vi "RampVoltagewithDDSv7.vi"() -> ()   [LabVIEW 2016]
uses:
  <vilib>/DAQmx/write.llb/DAQmx Write (Digital 1D Wfm NChan NSamp).vi
  <vilib>/DAQmx/write.llb/DAQmx Write (Analog 2D DBL NChan NSamp).vi
  <vilib>/DAQmx/create/channels.llb/DAQmx Create Channel (AO-Voltage-Basic).vi
  <vilib>/DAQmx/create/channels.llb/DAQmx Create Channel (DO-Digital Output).vi
  <vilib>/DAQmx/configure/timing.llb/DAQmx Timing (Sample Clock).vi
  <vilib>/DAQmx/configure/trigger.llb/DAQmx Start Trigger (Digital Edge).vi
  <vilib>/DAQmx/miscellaneous.llb/DAQmx Fill In Error Info.vi
  <vilib>/Waveform/DWDTOps.llb/DWDT Boolean Array to Digital.vi
  <vilib>/Waveform/DWDTOps.llb/DWDT Uncompress Digital.vi
  <vilib>/Waveform/DTblOps.llb/DTbl Digital to Analog.vi
  <resource>/objmgr/daqmx.rc
panel:
  in  "Reset Digital Outputs":bool
  in  "DDS Trigger delay (ms)":dbl step=0.01
  in  "DDS Trigger (Port 0 Line 1)":tag="Dev2/port0/line1"
  out "Digital Output":cluster{i32, dbl, dbl[][]}(graph)={0, 1e-05, [[5.0, 5.0, 5.0, 5.0, 5.0, 5.0, 5.0, 5.0, 5.0, 5.0, 5.0, 5.0, 5.0, 5.0, 5.0, 5.0, 5.0, 5.0, 5.0, 5.0, 5.0, 5.0, 5.0, 5.0, 5.0, 5.0, 5.0, 5.0, 5.0, 5.0, 5.0, 5.0, 5.0, 5.0, 5.0, 5.0, 5.0, 5.0, 5.0, 5.0, 5.0, 5.0, 5.0, 5.0, 5.0, 5.0, 5.0, 5.0, 5.0, 5.0, 5.0, 5.0, 5.0, 5.0, 5.0, 5.0, 5.0, 5.0, 5.0, 5.0, 5.0, 5.0, 5.0, 5.0, 5.0, 5.0, 5.0, 5.0, 5.0, 5.0, 5.0, 5.0, 5.0, 5.0, 5.0, 5.0, 5.0, 5.0, 5.0, 5.0, 5.0, 5.0, 5.0, 5.0, 5.0, 5.0, 5.0, 5.0, 5.0, 5.0, 5.0, 5.0, 5.0, 5.0, 5.0, 5.0, 5.0, 5.0, 5.0, 5.0, 0.0, 0.0, 0.0, 0.0, 0.0, 0.0, 0.0, 0.0, 0.0, 0.0, 0.0, 0.0, 0.0, 0.0, 0.0, 0.0, 0.0, 0.0, 0.0, 0.0, 0.0, 0.0, 0.0, 0.0, 0.0, 0.0, 0.0, 0.0, 0.0, 0.0, 0.0, 0.0, 0.0, 0.0, 0.0, 0.0, 0.0, 0.0, 0.0, 0.0, 0.0, 0.0, 0.0, 0.0, 0.0, 0.0, 0.0, 0.0, 0.0, 0.0, 0.0, 0.0, 0.0, 0.0, 0.0, 0.0, 0.0, 0.0, 0.0, 0.0, 0.0, 0.0, 0.0, 0.0, 0.0, 0.0, 0.0, 0.0, 0.0, 0.0, 0.0, 0.0, 0.0, 0.0, 0.0, 0.0, 0.0, 0.0, 0.0, 0.0, 0.0, 0.0, 0.0, 0.0, 0.0, 0.0, 0.0, 0.0, 0.0, 0.0, 0.0, 0.0, 0.0, 0.0, 0.0, 0.0, 0.0, 0.0, 0.0, 0.0, 0.0, 0.0, 0.0, 0.0, 0.0, 0.0, 0.0, 0.0, 0.0, 0.0, 0.0, 0.0, 0.0, 0.0, 0.0, 0.0, 0.0, 0.0, 0.0, 0.0, 0.0, 0.0, 0.0, 0.0, 0.0, 0.0, 0.0, 0.0, 0.0, 0.0, 0.0, 0.0, 0.0, 0.0, 0.0, 0.0, 0.0, 0.0, 0.0, 0.0, 0.0, 0.0, 0.0, 0.0, 0.0, 0.0, 0.0, 0.0, 0.0, 0.0, 0.0, 0.0, 0.0, 0.0, 0.0, 0.0, 0.0, 0.0, 0.0, 0.0, 0.0, 0.0, 0.0, 0.0, 0.0, 0.0, 0.0, 0.0, 0.0, 0.0, 0.0, 0.0, 0.0, 0.0, 0.0, 0.0, 0.0, 0.0, 0.0, 0.0, 0.0, 0.0, 0.0, 0.0, 0.0, 0.0, 0.0, 0.0, 0.0, 0.0, 0.0, 0.0, 0.0, 0.0, 0.0, 0.0, 0.0, 0.0, 0.0, 0.0, 5.0, 5.0, 5.0, 5.0, 5.0, 5.0, 5.0, 5.0, 5.0, 5.0, 5.0, 5.0, 5.0, 5.0, 5.0, 5.0, 5.0, 5.0, 5.0, 5.0, 5.0, 5.0, 5.0, 5.0, 5.0, 5.0, 5.0, 5.0, 5.0, 5.0, 5.0, 5.0, 5.0, 5.0, 5.0, 5.0, 5.0, 5.0, 5.0, 5.0, 5.0, 5.0, 5.0, 5.0, 5.0, 5.0, 5.0, 5.0, 5.0, 5.0, 5.0, 5.0, 5.0, 5.0, 5.0, 5.0, 5.0, 5.0, 5.0, 5.0, 5.0, 5.0, 5.0, 5.0, 5.0, 5.0, 5.0, 5.0, 5.0, 5.0, 5.0, 5.0, 5.0, 5.0, 5.0, 5.0, 5.0, 5.0, 5.0, 5.0, 5.0, 5.0, 5.0, 5.0, 5.0, 5.0, 5.0, 5.0, 5.0, 5.0, 5.0, 5.0, 5.0, 5.0, 5.0, 5.0, 5.0, 5.0, 5.0, 5.0, 5.0, 5.0, 5.0, 5.0, 5.0, 5.0, 5.0, 5.0, 5.0, 5.0, 5.0, 5.0, 5.0, 5.0, 5.0, 5.0, 5.0, 5.0, 5.0, 5.0, 5.0, 5.0, 5.0, 5.0, 5.0, 5.0, 5.0, 5.0, 5.0, 5.0, 5.0, 5.0, 5.0, 5.0, 5.0, 5.0, 5.0, 5.0, 5.0, 5.0, 5.0, 5.0, 5.0, 5.0, 5.0, 5.0, 5.0, 5.0, 5.0, 5.0, 5.0, 5.0, 5.0, 5.0, 5.0, 5.0, 5.0, 5.0, 5.0, 5.0, 5.0, 5.0, 5.0, 5.0, 5.0, 5.0, 5.0, 5.0, 5.0, 5.0, 5.0, 5.0, 5.0, 5.0, 5.0, 5.0, 5.0, 5.0, 5.0, 5.0, 5.0, 5.0, 5.0, 5.0, 5.0, 5.0, 5.0, 5.0, 5.0, 5.0, 5.0, 5.0, 5.0, 5.0, 5.0, 5.0, 5.0, 5.0, 5.0, 5.0, 0.0, 0.0, 0.0, 0.0, 0.0, 0.0, 0.0, 0.0, 0.0, 0.0, 0.0, 0.0, 0.0, 0.0, 0.0, 0.0, 0.0, 0.0, 0.0, 0.0, 0.0, 0.0, 0.0, 0.0, 0.0, 0.0, 0.0, 0.0, 0.0, 0.0, 0.0, 0.0, 0.0, 0.0, 0.0, 0.0, 0.0, 0.0, 0.0, 0.0, 0.0, 0.0, 0.0, 0.0, 0.0, 0.0, 0.0, 0.0, 0.0, 0.0, 0.0, 0.0, 0.0, 0.0, 0.0, 0.0, 0.0, 0.0, 0.0, 0.0, 0.0, 0.0, 0.0, 0.0, 0.0, 0.0, 0.0, 0.0, 0.0, 0.0, 0.0, 0.0, 0.0, 0.0, 0.0, 0.0, 0.0, 0.0, 0.0, 0.0, 0.0, 0.0, 0.0, 0.0, 0.0, 0.0, 0.0, 0.0, 0.0, 0.0, 0.0, 0.0, 0.0, 0.0, 0.0, 0.0, 0.0, 0.0, 0.0, 0.0, 0.0, 0.0, 0.0, 0.0, 0.0, 0.0, 0.0, 0.0, 0.0, 0.0, 0.0, 0.0, 0.0, 0.0, 0.0, 0.0, 0.0, 0.0, 0.0, 0.0, 0.0, 0.0, 0.0, 0.0, 0.0, 0.0, 0.0, 0.0, 0.0, 0.0, 0.0, 0.0, 0.0, 0.0, 0.0, 0.0, 0.0, 0.0, 0.0, 0.0, 0.0, 0.0, 0.0, 0.0, 0.0, 0.0, 0.0, 0.0, 0.0, 0.0, 0.0, 0.0, 0.0, 0.0, 0.0, 0.0, 0.0, 0.0, 0.0, 0.0, 0.0, 0.0, 0.0, 0.0, 0.0, 0.0, 0.0, 0.0, 0.0, 0.0, 0.0, 0.0, 0.0, 0.0, 0.0, 0.0, 0.0, 0.0, 0.0, 0.0, 0.0, 0.0, 0.0, 0.0, 0.0, 0.0, 0.0, 0.0, 0.0, 0.0, 0.0, 0.0, 0.0, 0.0, 0.0, 0.0, 0.0, 0.0, 0.0, 0.0, 5.0, 5.0, 5.0, 5.0, 5.0, 5.0, 5.0, 5.0, 5.0, 5.0, 5.0, 5.0, 5.0, 5.0, 5.0, 5.0, 5.0, 5.0, 5.0, 5.0, 5.0, 5.0, 5.0, 5.0, 5.0, 5.0, 5.0, 5.0, 5.0, 5.0, 5.0, 5.0, 5.0, 5.0, 5.0, 5.0, 5.0, 5.0, 5.0, 5.0, 5.0, 5.0, 5.0, 5.0, 5.0, 5.0, 5.0, 5.0, 5.0, 5.0, 5.0, 5.0, 5.0, 5.0, 5.0, 5.0, 5.0, 5.0, 5.0, 5.0, 5.0, 5.0, 5.0, 5.0, 5.0, 5.0, 5.0, 5.0, 5.0, 5.0, 5.0, 5.0, 5.0, 5.0, 5.0, 5.0, 5.0, 5.0, 5.0, 5.0, 5.0, 5.0, 5.0, 5.0, 5.0, 5.0, 5.0, 5.0, 5.0, 5.0, 5.0, 5.0, 5.0, 5.0, 5.0, 5.0, 5.0, 5.0, 5.0, 5.0, 5.0], [5.0, 5.0, 5.0, 5.0, 5.0, 5.0, 5.0, 5.0, 5.0, 5.0, 5.0, 5.0, 5.0, 5.0, 5.0, 5.0, 5.0, 5.0, 5.0, 5.0, 5.0, 5.0, 5.0, 5.0, 5.0, 5.0, 5.0, 5.0, 5.0, 5.0, 5.0, 5.0, 5.0, 5.0, 5.0, 5.0, 5.0, 5.0, 5.0, 5.0, 5.0, 5.0, 5.0, 5.0, 5.0, 5.0, 5.0, 5.0, 5.0, 5.0, 5.0, 5.0, 5.0, 5.0, 5.0, 5.0, 5.0, 5.0, 5.0, 5.0, 5.0, 5.0, 5.0, 5.0, 5.0, 5.0, 5.0, 5.0, 5.0, 5.0, 5.0, 5.0, 5.0, 5.0, 5.0, 5.0, 5.0, 5.0, 5.0, 5.0, 5.0, 5.0, 5.0, 5.0, 5.0, 5.0, 5.0, 5.0, 5.0, 5.0, 5.0, 5.0, 5.0, 5.0, 5.0, 5.0, 5.0, 5.0, 5.0, 5.0, 0.0, 0.0, 0.0, 0.0, 0.0, 0.0, 0.0, 0.0, 0.0, 0.0, 0.0, 0.0, 0.0, 0.0, 0.0, 0.0, 0.0, 0.0, 0.0, 0.0, 0.0, 0.0, 0.0, 0.0, 0.0, 0.0, 0.0, 0.0, 0.0, 0.0, 0.0, 0.0, 0.0, 0.0, 0.0, 0.0, 0.0, 0.0, 0.0, 0.0, 0.0, 0.0, 0.0, 0.0, 0.0, 0.0, 0.0, 0.0, 0.0, 0.0, 0.0, 0.0, 0.0, 0.0, 0.0, 0.0, 0.0, 0.0, 0.0, 0.0, 0.0, 0.0, 0.0, 0.0, 0.0, 0.0, 0.0, 0.0, 0.0, 0.0, 0.0, 0.0, 0.0, 0.0, 0.0, 0.0, 0.0, 0.0, 0.0, 0.0, 0.0, 0.0, 0.0, 0.0, 0.0, 0.0, 0.0, 0.0, 0.0, 0.0, 0.0, 0.0, 0.0, 0.0, 0.0, 0.0, 0.0, 0.0, 0.0, 0.0, 0.0, 0.0, 0.0, 0.0, 0.0, 0.0, 0.0, 0.0, 0.0, 0.0, 0.0, 0.0, 0.0, 0.0, 0.0, 0.0, 0.0, 0.0, 0.0, 0.0, 0.0, 0.0, 0.0, 0.0, 0.0, 0.0, 0.0, 0.0, 0.0, 0.0, 0.0, 0.0, 0.0, 0.0, 0.0, 0.0, 0.0, 0.0, 0.0, 0.0, 0.0, 0.0, 0.0, 0.0, 0.0, 0.0, 0.0, 0.0, 0.0, 0.0, 0.0, 0.0, 0.0, 0.0, 0.0, 0.0, 0.0, 0.0, 0.0, 0.0, 0.0, 0.0, 0.0, 0.0, 0.0, 0.0, 0.0, 0.0, 0.0, 0.0, 0.0, 0.0, 0.0, 0.0, 0.0, 0.0, 0.0, 0.0, 0.0, 0.0, 0.0, 0.0, 0.0, 0.0, 0.0, 0.0, 0.0, 0.0, 0.0, 0.0, 0.0, 0.0, 0.0, 0.0, 0.0, 0.0, 0.0, 0.0, 0.0, 0.0, 0.0, 0.0, 0.0, 0.0, 0.0, 0.0, 0.0, 0.0, 0.0, 0.0, 0.0, 0.0, 0.0, 0.0, 0.0, 0.0, 0.0, 0.0, 0.0, 0.0, 0.0, 0.0, 0.0, 0.0, 0.0, 0.0, 0.0, 0.0, 0.0, 0.0, 0.0, 0.0, 0.0, 0.0, 0.0, 0.0, 0.0, 0.0, 0.0, 0.0, 0.0, 0.0, 0.0, 0.0, 0.0, 0.0, 0.0, 0.0, 0.0, 0.0, 0.0, 0.0, 0.0, 0.0, 0.0, 0.0, 0.0, 0.0, 0.0, 0.0, 0.0, 0.0, 0.0, 0.0, 0.0, 0.0, 0.0, 0.0, 0.0, 0.0, 0.0, 0.0, 0.0, 0.0, 0.0, 0.0, 0.0, 0.0, 0.0, 0.0, 0.0, 0.0, 0.0, 0.0, 0.0, 0.0, 0.0, 0.0, 0.0, 0.0, 0.0, 0.0, 0.0, 0.0, 0.0, 0.0, 0.0, 0.0, 0.0, 0.0, 0.0, 0.0, 0.0, 0.0, 0.0, 0.0, 0.0, 0.0, 0.0, 0.0, 0.0, 0.0, 0.0, 0.0, 0.0, 0.0, 0.0, 0.0, 0.0, 0.0, 0.0, 0.0, 0.0, 0.0, 0.0, 0.0, 0.0, 0.0, 0.0, 0.0, 0.0, 0.0, 0.0, 0.0, 0.0, 0.0, 0.0, 0.0, 0.0, 0.0, 0.0, 0.0, 0.0, 0.0, 0.0, 0.0, 0.0, 0.0, 0.0, 0.0, 0.0, 0.0, 0.0, 0.0, 0.0, 0.0, 0.0, 0.0, 0.0, 0.0, 0.0, 0.0, 0.0, 0.0, 0.0, 0.0, 0.0, 0.0, 0.0, 0.0, 0.0, 0.0, 0.0, 0.0, 0.0, 0.0, 0.0, 0.0, 0.0, 0.0, 0.0, 0.0, 0.0, 0.0, 0.0, 0.0, 0.0, 0.0, 0.0, 0.0, 0.0, 0.0, 0.0, 0.0, 0.0, 0.0, 0.0, 0.0, 0.0, 0.0, 0.0, 0.0, 0.0, 0.0, 0.0, 0.0, 0.0, 0.0, 0.0, 0.0, 0.0, 0.0, 0.0, 0.0, 0.0, 0.0, 0.0, 0.0, 0.0, 0.0, 0.0, 0.0, 0.0, 0.0, 0.0, 0.0, 0.0, 0.0, 0.0, 0.0, 0.0, 0.0, 0.0, 0.0, 0.0, 0.0, 0.0, 0.0, 0.0, 0.0, 0.0, 0.0, 0.0, 0.0, 0.0, 0.0, 0.0, 0.0, 0.0, 0.0, 0.0, 0.0, 0.0, 0.0, 0.0, 0.0, 0.0, 0.0, 0.0, 0.0, 0.0, 0.0, 0.0, 0.0, 0.0, 0.0, 0.0, 0.0, 0.0, 0.0, 0.0, 0.0, 0.0, 0.0, 0.0, 0.0, 0.0, 0.0, 0.0, 0.0, 0.0, 0.0, 0.0, 0.0, 0.0, 0.0, 0.0, 0.0, 0.0, 0.0, 0.0, 0.0, 0.0, 0.0, 0.0, 0.0, 0.0, 0.0, 0.0, 0.0, 0.0, 0.0, 0.0, 0.0, 0.0, 0.0, 0.0, 0.0, 0.0, 0.0, 0.0, 0.0, 0.0, 0.0, 0.0, 0.0, 0.0, 0.0, 0.0, 0.0, 0.0, 0.0, 0.0, 0.0, 0.0, 0.0, 0.0, 0.0, 0.0, 0.0, 0.0, 0.0, 0.0, 0.0, 0.0, 0.0, 0.0, 0.0, 0.0, 0.0, 0.0, 0.0, 0.0, 0.0, 0.0, 0.0, 0.0, 0.0, 0.0, 0.0, 0.0, 0.0, 0.0, 0.0, 0.0, 0.0, 0.0, 0.0, 0.0, 0.0, 0.0, 0.0, 0.0, 0.0, 0.0, 0.0, 0.0, 0.0, 0.0, 0.0, 0.0, 0.0, 0.0, 0.0, 0.0, 0.0, 0.0, 0.0, 0.0, 0.0, 0.0, 0.0, 0.0, 0.0, 0.0, 0.0, 0.0, 0.0, 0.0, 0.0, 0.0, 0.0, 0.0, 0.0, 0.0, 0.0, 0.0, 0.0, 0.0, 0.0, 0.0, 0.0, 0.0, 0.0, 0.0, 0.0, 0.0, 0.0, 0.0, 0.0, 0.0, 0.0, 0.0, 0.0, 0.0, 0.0, 0.0, 0.0, 0.0, 0.0, 0.0, 0.0, 0.0, 0.0, 0.0, 0.0, 0.0, 0.0, 0.0, 0.0, 0.0, 0.0, 0.0, 0.0, 0.0, 0.0, 0.0, 0.0, 0.0, 0.0, 0.0, 0.0, 0.0, 0.0, 0.0, 0.0, 0.0, 0.0, 0.0, 0.0, 0.0, 0.0, 0.0, 0.0, 0.0, 0.0, 0.0, 0.0, 0.0, 0.0, 0.0, 0.0, 0.0, 0.0, 0.0, 0.0, 0.0, 0.0, 0.0, 0.0, 0.0, 0.0, 0.0, 0.0, 0.0, 0.0, 0.0, 0.0, 0.0, 0.0, 0.0, 0.0, 0.0, 0.0, 0.0, 0.0, 0.0, 0.0, 0.0, 0.0, 0.0, 0.0, 0.0, 0.0, 0.0, 0.0, 0.0, 0.0, 0.0, 0.0, 5.0]]}
  out "Analog Outputs":cluster{i32, dbl, dbl[][]}(graph)={0, 4e-06, array4x2001[8004 elements]}
  in  "High Gain Switch (Port 0 Line 0)":tag="Dev2/port0/line0"
  in  "Ramp to high gain \ndelay (ms)":dbl step=0.01
  in  "error in 2":errorcluster caption="error in"
  in  "ao3 ramp amplitude (V)":dbl=0.4
  in  "ao2 ramp amplitude (V)":dbl=0.3
  in  "ao1 ramp amplitude (V)":dbl=0.2
  in  "SolsTiS 2 - Fast Piezo (ao3)":tag="Dev2/ao3"
  in  "SolsTiS 2 - Slow Piezo (ao2)":tag="Dev2/ao2"
  out "size(s)":i32=2001
  in  "Trigger delay NI (ms)":dbl=1.0
  in  "Trigger Input (PFI0)":tag="/Dev2/PFI0"
  in  "SolsTiS 1 - Fast Piezo (ao1)":tag="Dev2/ao1"
  in  "SolsTiS 1 - Slow Piezo (ao0)":tag="Dev2/ao0"
  in  "Plateau duration (ms)":dbl=2.0 step=0.01
  in  "Ramp duration (ms)":dbl=2.0 step=0.01
  in  "ao0 ramp amplitude (V)":dbl=1.0 step=0.001
  in  "error in":errorcluster
  # "MAGIS LASER SYSTEM\nChirp Control"
  # "Ramp Definition"
  # "Output Monitor"
  # "Channel Definition"
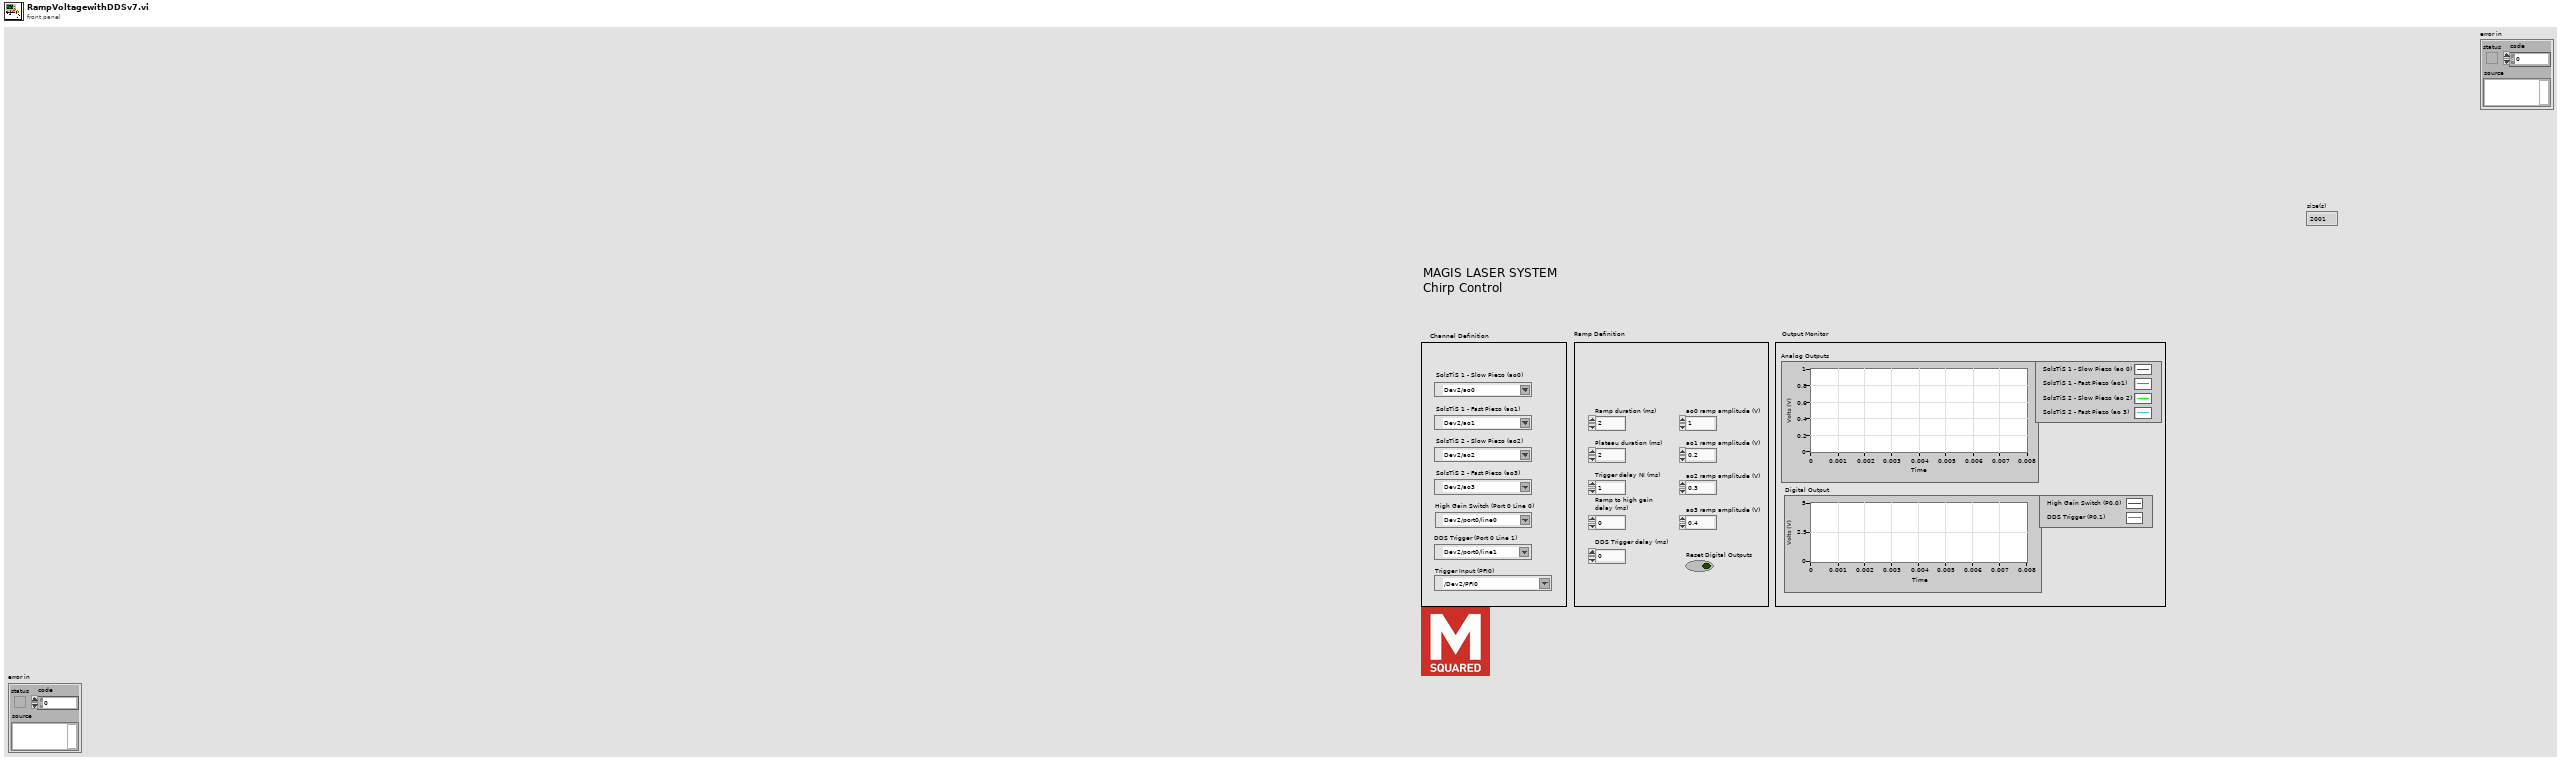
[diagram p1: front panel]
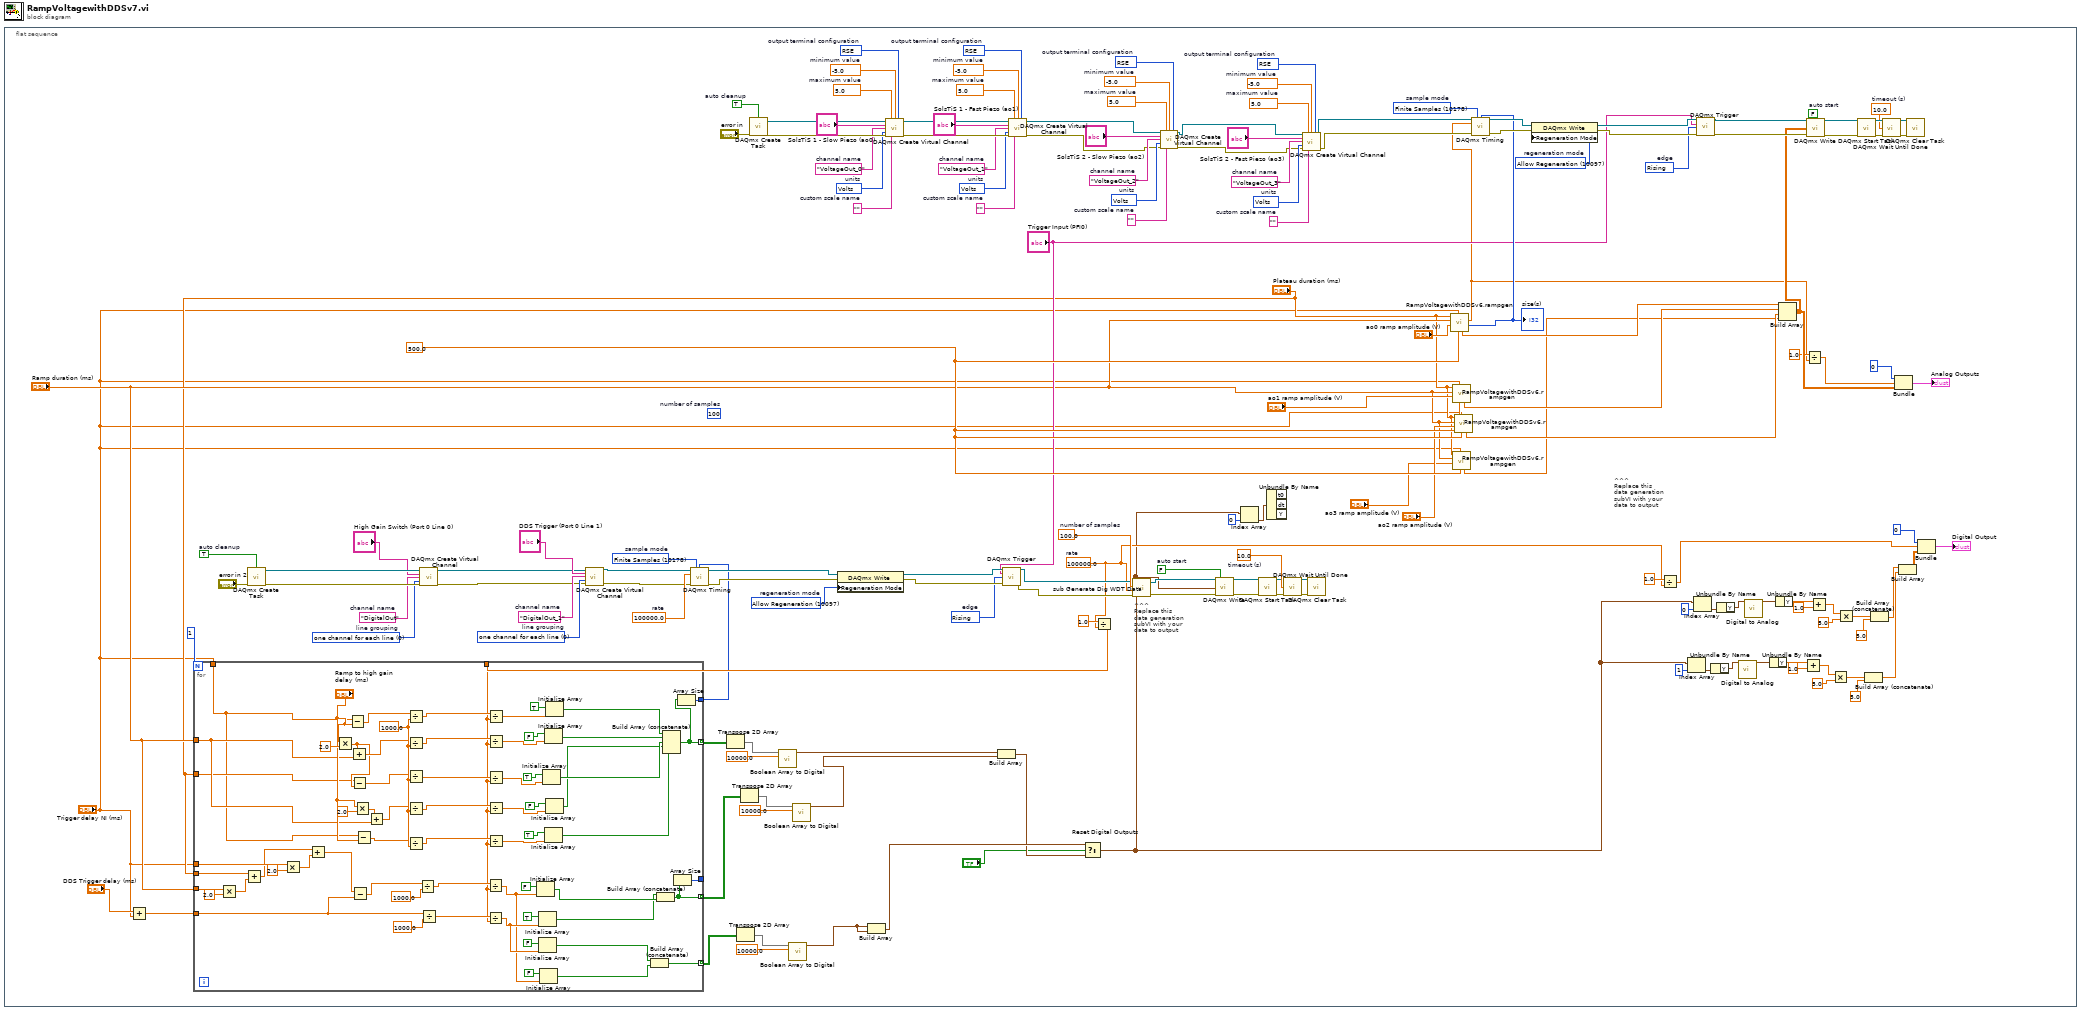
[diagram p0: block diagram]
diagram:
  n1 = flat-sequence {
    frame #0 {
      w36 = 0 items=["one channel for each line", "one channel for all lines"]  # line grouping
      w35 = "DigitalOut_1"  # channel name
      w104 = 500.0 ("No of samples in ramp (500 or less)")
      w71 = 10280 items=["Rising"=10280, "Falling"=10171]  # edge
      w73 = 10097 items=["Allow Regeneration"=10097, "Do Not Allow Regeneration"=10158]  # regeneration mode
      w76 = 10178 items=["Finite Samples"=10178, "Continuous Samples"=10123, "Hardware Timed Single Point"=12522]  # sample mode
      (unwired) 100  # number of samples
      w77 = 100000.0  # rate
      w80 = 0 items=["one channel for each line", "one channel for all lines"]  # line grouping
      w79 = "DigitalOut"  # channel name
      w82 = TRUE  # auto cleanup
      w97 = 10.0  # timeout (s)
      w45 = 100000.0  # rate
      w90 = 100.0  # number of samples
      w87 = FALSE  # auto start
      w111 = 10083 items=["Default"=-1, "RSE"=10083, "Differential"=10106, "Pseudodifferential"=12529]  # output terminal configuration
      w112 = 10348 items=["Volts"=10348, "From Custom Scale"=10065]  # units
      w113 = "VoltageOut_3"  # channel name
      w114 = ""  # custom scale name
      w115 = -5.0  # minimum value
      w116 = 5.0  # maximum value
      w120 = 10083 items=["Default"=-1, "RSE"=10083, "Differential"=10106, "Pseudodifferential"=12529]  # output terminal configuration
      w121 = 10348 items=["Volts"=10348, "From Custom Scale"=10065]  # units
      w122 = "VoltageOut_2"  # channel name
      w123 = ""  # custom scale name
      w124 = -5.0  # minimum value
      w125 = 5.0  # maximum value
      w132 = 10280 items=["Rising"=10280, "Falling"=10171]  # edge
      w134 = 10097 items=["Allow Regeneration"=10097, "Do Not Allow Regeneration"=10158]  # regeneration mode
      w137 = 10178 items=["Finite Samples"=10178, "Continuous Samples"=10123, "Hardware Timed Single Point"=12522]  # sample mode
      w139 = 10083 items=["Default"=-1, "RSE"=10083, "Differential"=10106, "Pseudodifferential"=12529]  # output terminal configuration
      w140 = 10348 items=["Volts"=10348, "From Custom Scale"=10065]  # units
      w141 = "VoltageOut_1"  # channel name
      w142 = ""  # custom scale name
      w143 = -5.0  # minimum value
      w144 = 5.0  # maximum value
      w146 = 10083 items=["Default"=-1, "RSE"=10083, "Differential"=10106, "Pseudodifferential"=12529]  # output terminal configuration
      w147 = 10348 items=["Volts"=10348, "From Custom Scale"=10065]  # units
      w148 = "VoltageOut_0"  # channel name
      w150 = ""  # custom scale name
      w151 = -5.0  # minimum value
      w152 = 5.0  # maximum value
      w154 = TRUE  # auto cleanup
      w160 = 10.0  # timeout (s)
      w164 = FALSE  # auto start
      # "^^^\nReplace this\ndata generation\nsubVI with your\ndata to output"
      # "^^^\nReplace this\ndata generation\nsubVI with your\ndata to output"
      n2 = Add(x="DDS Trigger delay (ms)", y="Trigger delay NI (ms)") -> (x+y=w27:dbl)
      n3 = call <vilib>:"DAQmx Create Task.vi"("auto cleanup"=w82, "error in"="error in 2") -> ("task out"=w81:refnum<k21>, "error out"=w83:errorcluster)  [unwired: 12 in]
      n4 = call-poly <vilib>:"DAQmx Create Virtual Channel.vi"("task in"=w81, "lines"="High Gain Switch (Port 0 Line 0)", "name to assign"=w79, "line grouping"=w80, "error in"=w83) -> ("task out"=w30:refnum<k21>, "error out"=w33:errorcluster)  [unwired: 9 in]
      n5 = call-poly <vilib>:"DAQmx Create Virtual Channel.vi"("task in"=w30, "lines"="DDS Trigger (Port 0 Line 1)", "name to assign"=w35, "line grouping"=w36, "error in"=w33) -> ("task out"=w32:refnum<k21>, "error out"=w31:errorcluster)  [unwired: 9 in]
      n6 = call <vilib>:"DAQmx Create Task.vi"("auto cleanup"=w154, "error in"="error in") -> ("task out"=w153:refnum<k21>, "error out"=w155:errorcluster)  [unwired: 12 in]
      n7 = call-poly <vilib>:"DAQmx Create Virtual Channel.vi"("task in"=w153, "maximum value"=w152, "minimum value"=w151, "output terminal configuration"=w146, "physical channels"="SolsTiS 1 - Slow Piezo (ao0)", "name to assign"=w148, "units"=w147, "error in"=w155, "custom scale name"=w150) -> ("task out"=w145:refnum<k21>, "error out"=w149:errorcluster)  [unwired: 5 in]
      n8 = call-poly <vilib>:"DAQmx Create Virtual Channel.vi"("task in"=w145, "maximum value"=w144, "minimum value"=w143, "output terminal configuration"=w139, "physical channels"="SolsTiS 1 - Fast Piezo (ao1)", "name to assign"=w141, "units"=w140, "error in"=w149, "custom scale name"=w142) -> ("task out"=w118:refnum<k21>, "error out"=w117:errorcluster)  [unwired: 5 in]
      n9 = Divide(x=1.0, y=w45) -> (x/y=w67:dbl)
      n10 = for {
        N: 1 -> [_]
        tunnel: w67 -> [w181]
        tunnel: [w208] -> w64 mode=indexing
        tunnel: [w207] -> w63
        tunnel: "Ramp duration (ms)" -> [w196]
        tunnel: "Plateau duration (ms)" -> [w195]
        tunnel: "Trigger delay NI (ms)" -> [w194]
        tunnel: w27 -> [w187]
        tunnel: "Ramp duration (ms)" -> [w191]
        tunnel: "Plateau duration (ms)" -> [w188]
        tunnel: [w178] -> _
        tunnel: "Trigger delay NI (ms)" -> [w175]
        tunnel: [w172] -> w21 mode=indexing
        tunnel: [w165] -> w17 mode=indexing
        w227 = 1000.0
        n11 = Multiply(x=w191, y=2.0) -> (x*y=w189:dbl)
        n12 = Add(x=w188, y=w189) -> (x+y=w174:dbl)
        n13 = Multiply(x=w175, y=2.0) -> (x*y=w176:dbl)
        n14 = Add(x=w174, y=w176) -> (x+y=w173:dbl)
        n15 = Multiply(x="Ramp to high gain \ndelay (ms)", y=2.0) -> (x*y=w203:dbl)
        n16 = Subtract(x=w194, y="Ramp to high gain \ndelay (ms)") -> (x-y=w206:dbl)
        n17 = Add(x=w203, y=w196) -> (x+y=w204:dbl)
        n18 = Subtract(x=w195, y=w203) -> (x-y=w202:dbl)
        n19 = Subtract(x=w173, y=w187) -> (x-y=w184:dbl)
        n20 = Multiply(x="Ramp to high gain \ndelay (ms)", y=2.0) -> (x*y=w200:dbl)
        n21 = Subtract(x=w194, y="Ramp to high gain \ndelay (ms)") -> (x-y=w197:dbl)
        n22 = Add(x=w200, y=w196) -> (x+y=w199:dbl)
        n23 = Divide(x=w206, y=w227) -> (x/y=w226:dbl)
        n24 = Divide(x=w204, y=w227) -> (x/y=w225:dbl)
        n25 = Divide(x=w202, y=w227) -> (x/y=w224:dbl)
        n26 = Divide(x=w199, y=w227) -> (x/y=w223:dbl)
        n27 = Divide(x=w197, y=w227) -> (x/y=w222:dbl)
        n28 = Divide(x=w184, y=1000.0) -> (x/y=w183:dbl)
        n29 = Divide(x=w187, y=1000.0) -> (x/y=w182:dbl)
        n30 = Divide(x=w183, y=w181) -> (x/y=w168:dbl)
        n31 = Divide(x=w182, y=w181) -> (x/y=w169:dbl)
        n32 = Divide(x=w226, y=w181) -> (x/y=w218:dbl)
        n33 = Divide(x=w225, y=w181) -> (x/y=w217:dbl)
        n34 = Divide(x=w224, y=w181) -> (x/y=w216:dbl)
        n35 = Divide(x=w223, y=w181) -> (x/y=w215:dbl)
        n36 = Divide(x=w222, y=w181) -> (x/y=w214:dbl)
        n37 = Initialize Array(FALSE, w168) -> (w180:bool[])
        n38 = Initialize Array(TRUE, w169) -> (w179:bool[])
        n39 = Initialize Array(FALSE, w169) -> (w167:bool[])
        n40 = Initialize Array(FALSE, w168) -> (w166:bool[])
        n41 = Initialize Array(TRUE, w216) -> (w211:bool[])
        n42 = Initialize Array(FALSE, w217) -> (w212:bool[])
        n43 = Initialize Array(TRUE, w214) -> (w209:bool[])
        n44 = Initialize Array(TRUE, w218) -> (w213:bool[])
        n45 = Initialize Array(FALSE, w215) -> (w210:bool[])
        n46 = Build Array (concatenate)(w167, w166) -> (w165:bool[])
        n47 = Build Array (concatenate)(w179, w180) -> (w172:bool[])
        n48 = Build Array (concatenate)(w213, w212, w211, w210, w209) -> (w208:bool[])
        n49 = Array Size(array=w172) -> (size(s)=w178:i32)
        n50 = Array Size(array=w208) -> (size(s)=w207:i32)
      }
      n51 = call-poly <vilib>:"DAQmx Timing.vi"("task/channels in"=w32, "sample mode"=w76, "samples per channel"=w63, "rate"=w77, "error in"=w31) -> ("task out"=w75:refnum<k21>, "error out"=w78:errorcluster)  [unwired: 9 in]
      n52 = Transpose 2D Array(2D array=w64) -> (transposed array=w65:bool[][])
      n53 = Transpose 2D Array(2D array=w17) -> (transposed array=w18:bool[][])
      n54 = Transpose 2D Array(2D array=w21) -> (transposed array=w22:bool[][])
      n55 = call-poly <vilib>:"Boolean Array to Digital.vi"("sample rate"=10000.0, "boolean array"=w65) -> ("digital waveform"=w29:digitalwaveform)  [unwired: 8 in, 1 out]
      n56 = call-poly <vilib>:"Boolean Array to Digital.vi"("sample rate"=10000.0, "boolean array"=w18) -> ("digital waveform"=w16:digitalwaveform)  [unwired: 8 in, 1 out]
      n57 = call-poly <vilib>:"Boolean Array to Digital.vi"("sample rate"=10000.0, "boolean array"=w22) -> ("digital waveform"=w20:digitalwaveform)  [unwired: 8 in, 1 out]
      n58 = property class="DAQmx Write"(reference=w75, error in=w78, "Regeneration Mode"=w73) -> (reference out=w72:refnum<k21>, error out=w74:errorcluster)
      n59 = Build Array(w16, w16) -> (w15:digitalwaveform[])
      n60 = Build Array(w29, w20) -> (w14:digitalwaveform[])
      n61 = call-poly <vilib>:"DAQmx Trigger.vi"("task/channels in"=w72, "source"="Trigger Input (PFI0)", "edge"=w71, "error in"=w74) -> ("task out"=w70:refnum<k21>, "error out"=w69:errorcluster)  [unwired: 10 in]
      n62 = Select(t=w15, s="Reset Digital Outputs", f=w14) -> (s? t:f=w2:digitalwaveform[])
      n63 = call <vilib>:"sub Generate Dig WDT Data.vi"("task in"=w70, "number of samples"=w90, "update rate"=w45, "error in"=w69) -> ("task out"=w89:refnum<k21>, "error out"=w88:errorcluster)  [unwired: 1 in, 1 out]
      n64 = call-poly <vilib>:"DAQmx Create Virtual Channel.vi"("task in"=w118, "maximum value"=w125, "minimum value"=w124, "output terminal configuration"=w120, "physical channels"="SolsTiS 2 - Slow Piezo (ao2)", "name to assign"=w122, "units"=w121, "error in"=w117, "custom scale name"=w123) -> ("task out"=w109:refnum<k21>, "error out"=w108:errorcluster)  [unwired: 5 in]
      n65 = call-poly <vilib>:"DAQmx Write.vi"("task/channels in"=w89, "auto start"=w87, "data"=w2, "error in"=w88) -> ("task out"=w94:refnum<k21>, "error out"=w95:errorcluster)  [unwired: 9 in, 1 out]
      n66 = Index Array(array=w2, index=0) -> (element=w85:digitalwaveform)
      n67 = call <vilib>:"DAQmx Start Task.vi"("task/channels in"=w94, "error in"=w95) -> ("task out"=w91:refnum<k21>, "error out"=w92:errorcluster)  [unwired: 12 in]
      n68 = Unbundle By Name(w85) -> ()  [unwired: 3 out]
      n69 = call <vilib>:"DAQmx Wait Until Done.vi"("task/channels in"=w91, "timeout (sec)"=w97, "error in"=w92) -> ("task out"=w96:refnum<k21>, "error out"=w93:errorcluster)  [unwired: 11 in]
      n70 = call-poly <vilib>:"DAQmx Create Virtual Channel.vi"("task in"=w109, "maximum value"=w116, "minimum value"=w115, "output terminal configuration"=w111, "physical channels"="SolsTiS 2 - Fast Piezo (ao3)", "name to assign"=w113, "units"=w112, "error in"=w108, "custom scale name"=w114) -> ("task out"=w106:refnum<k21>, "error out"=w107:errorcluster)  [unwired: 5 in]
      n71 = call <vilib>:"DAQmx Clear Task.vi"("task in"=w96, "error in"=w93) -> ()  [unwired: 13 in, 1 out]
      n72 = call "RampVoltagewithDDSv6,rampgen.vi"("No of samples in ramp"=w104, "Trigger delay NI (ms)"="Trigger delay NI (ms)", "Ramp Amplitude (V)}"="ao0 ramp amplitude (V)", "Ramp duration (ms)"="Ramp duration (ms)", "Plateau duration (ms)"="Plateau duration (ms)") -> ("Numeric 2"=w128:i32, "Numeric"=w48:dbl, "Array"=w105:dbl[])  [unwired: 3 in, 1 out]
      "size(s)" <- w128
      n73 = call "RampVoltagewithDDSv6,rampgen.vi"("No of samples in ramp"=w104, "Trigger delay NI (ms)"="Trigger delay NI (ms)", "Ramp Amplitude (V)}"="ao1 ramp amplitude (V)", "Ramp duration (ms)"="Ramp duration (ms)", "Plateau duration (ms)"="Plateau duration (ms)") -> ("Array"=w100:dbl[])  [unwired: 3 in, 3 out]
      n74 = call "RampVoltagewithDDSv6,rampgen.vi"("No of samples in ramp"=w104, "Trigger delay NI (ms)"="Trigger delay NI (ms)", "Ramp Amplitude (V)}"="ao3 ramp amplitude (V)", "Ramp duration (ms)"="Ramp duration (ms)", "Plateau duration (ms)"="Plateau duration (ms)") -> ("Array"=w98:dbl[])  [unwired: 3 in, 3 out]
      n75 = call "RampVoltagewithDDSv6,rampgen.vi"("No of samples in ramp"=w104, "Trigger delay NI (ms)"="Trigger delay NI (ms)", "Ramp Amplitude (V)}"="ao2 ramp amplitude (V)", "Ramp duration (ms)"="Ramp duration (ms)", "Plateau duration (ms)"="Plateau duration (ms)") -> ("Array"=w99:dbl[])  [unwired: 3 in, 3 out]
      n76 = call-poly <vilib>:"DAQmx Timing.vi"("task/channels in"=w106, "sample mode"=w137, "samples per channel"=w128, "rate"=w48, "error in"=w107) -> ("task out"=w136:refnum<k21>, "error out"=w138:errorcluster)  [unwired: 9 in]
      n77 = property class="DAQmx Write"(reference=w136, error in=w138, "Regeneration Mode"=w134) -> (reference out=w133:refnum<k21>, error out=w135:errorcluster)
      n78 = Divide(x=1.0, y=w45) -> (x/y=w44:dbl)
      n79 = Index Array(array=w2, index=1) -> (element=w11:digitalwaveform)
      n80 = Index Array(array=w2, index=0) -> (element=w55:digitalwaveform)
      n81 = call-poly <vilib>:"DAQmx Trigger.vi"("task/channels in"=w133, "source"="Trigger Input (PFI0)", "edge"=w132, "error in"=w135) -> ("task out"=w130:refnum<k21>, "error out"=w129:errorcluster)  [unwired: 10 in]
      n82 = Unbundle By Name(w11) -> ("Y"=w10:digitaldata)
      n83 = Unbundle By Name(w55) -> ("Y"=w54:digitaldata)
      n84 = call-poly <vilib>:"Digital to Analog.vi"("digital table"=w10) -> ("analog waveform"=w9:waveform(dbl))  [unwired: 7 in, 3 out]
      n85 = call-poly <vilib>:"Digital to Analog.vi"("digital table"=w54) -> ("analog waveform"=w53:waveform(dbl))  [unwired: 7 in, 3 out]
      n86 = Unbundle By Name(w9) -> ("Y"=w7:dbl[])
      n87 = Unbundle By Name(w53) -> ("Y"=w42:dbl[])
      n88 = Build Array(w105, w100, w99, w98) -> (w59:dbl[][])
      n89 = Add(x=w7, y=1.0) -> (x+y=w6:dbl[])
      n90 = Divide(x=1.0, y=w48) -> (x/y=w47:dbl)
      n91 = call-poly <vilib>:"DAQmx Write.vi"("task/channels in"=w130, "auto start"=w164, "data"=w59, "error in"=w129) -> ("task out"=w159:refnum<k21>, "error out"=w158:errorcluster)  [unwired: 9 in, 1 out]
      n92 = Add(x=w42, y=1.0) -> (x+y=w41:dbl[])
      n93 = Multiply(x=w6, y=5.0) -> (x*y=w4:dbl[])
      n94 = Multiply(x=w41, y=5.0) -> (x*y=w39:dbl[])
      n95 = call <vilib>:"DAQmx Start Task.vi"("task/channels in"=w159, "error in"=w158) -> ("task out"=w163:refnum<k21>, "error out"=w162:errorcluster)  [unwired: 12 in]
      n96 = Build Array (concatenate)(w4, 5.0 ("y")) -> (w1:dbl[])
      n97 = Build Array (concatenate)(w39, 5.0 ("y")) -> (w37:dbl[])
      n98 = call <vilib>:"DAQmx Wait Until Done.vi"("task/channels in"=w163, "timeout (sec)"=w160, "error in"=w162) -> ("task out"=w157:refnum<k21>, "error out"=w161:errorcluster)  [unwired: 11 in]
      n99 = Bundle(0, w47, w59) -> (→"Analog Outputs":cluster{i32, dbl, dbl[][]})  [unwired: 1 in]
      n100 = Build Array(w37, w1) -> (w50:dbl[][])
      n101 = call <vilib>:"DAQmx Clear Task.vi"("task in"=w157, "error in"=w161) -> ()  [unwired: 13 in, 1 out]
      n102 = Bundle(0, w44, w50) -> (→"Digital Output":cluster{i32, dbl, dbl[][]})  [unwired: 1 in]
    }
  }
